vi "RS232_Write-Read String.vi"(4 "Flow Control":u16(ring) items=["None"=0, "RTS-CTS"=256, "DTR-DSR"=512, "XOn-XOff"=1024], 5 "Stop Bits":u8(ring) items=["FT_STOP_BITS_1"=0, "FT_STOP_BITS_2"=2], 6 "Parity":u8(ring) items=["FT_PARITY_NONE", "FT_PARITY_ODD", "FT_PARITY_EVEN", "FT_PARITY_MARK", "FT_PARITY_SPACE"], 7 "Word Length":u8(ring)=8 items=["FT_BITS_7"=7, "FT_BITS_8"=8], 8 "Read Delay (ms)":u32=100, 9 "Write Buffer":string, 10 "Baud Rate":u32=115200, 11 "Device Description":string="TTL232RG-3V3_Application") -> (0 "Bytes Written":u32, 2 "Bytes Read":u32, 3 "Read Buffer Out":string)   [LabVIEW 2018]
panel:
  out "Ok?":bool
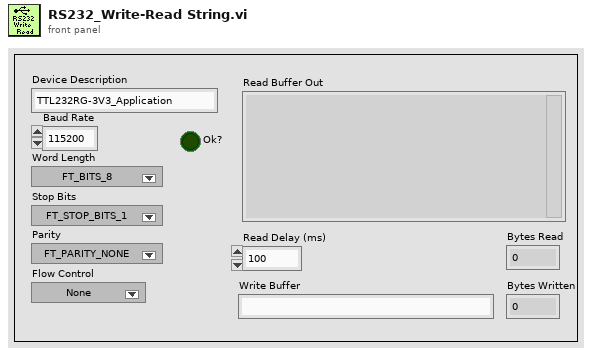
[diagram p1: front panel]
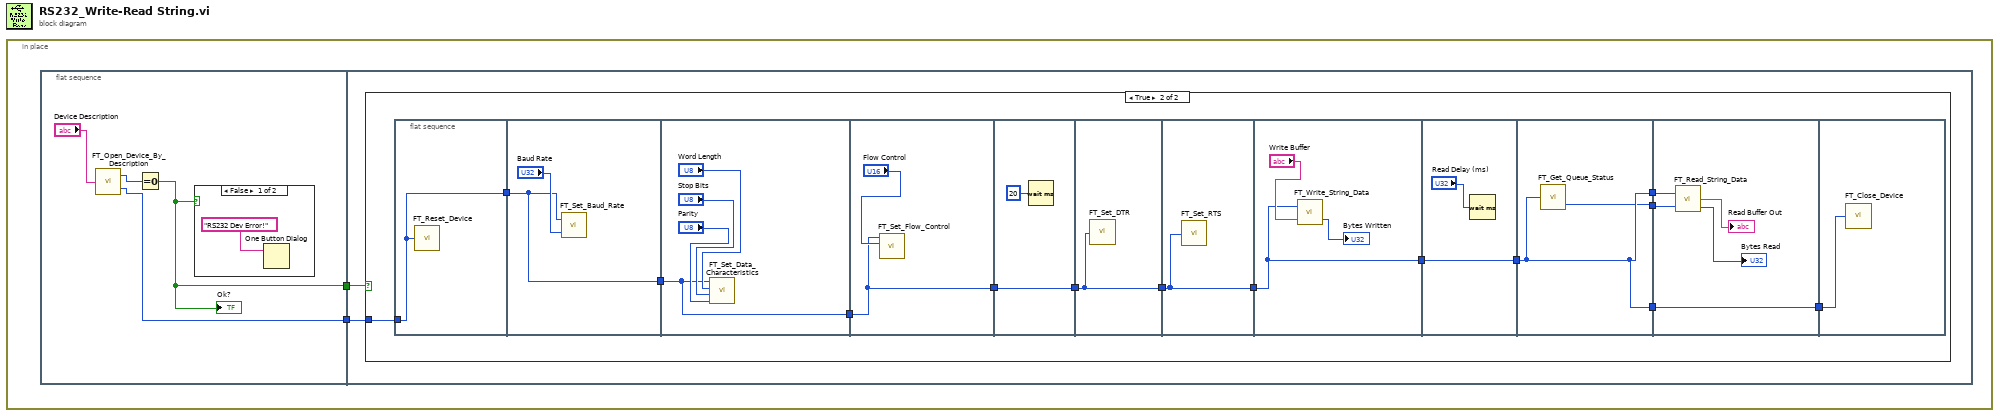
[diagram p0: block diagram]
diagram:
  n1 = in-place {
    n2 = flat-sequence {
      tunnel: [w5] -> w2
      tunnel: [w3] -> w1
      tunnel: w2 -> [w9]
      tunnel: w1 -> [w8]
      frame #0 {
        n3 = call "FT_Open_Device_By_Description.vi"("Device Description"="Device Description") -> ("FT_Status"=w4:u32, "Handle"=w3:u32)
        n4 = Equal To 0?(x=w4) -> (x = 0?=w5:bool)
        "Ok?" <- w5
        n5 = case shown="False" w5 {
          frame False {
            n6 = One Button Dialog(message="RS232 Dev Error!") -> ()  [unwired: 1 in, 1 out]
          }
          frame True {
          }
        }
      }
      frame #1 {
        n7 = case shown="True" w9 {
          tunnel: w8 -> [_ w14]
          frame False {
          }
          frame True {
            n8 = flat-sequence {
              tunnel: [w24] -> w23
              tunnel: w14 -> [w24]
              tunnel: w23 -> [w25]
              tunnel: [w25] -> w22
              tunnel: w22 -> [w27]
              tunnel: [w27] -> w21
              tunnel: w21 -> [w31]
              tunnel: [w31] -> w13
              tunnel: w13 -> [w34]
              tunnel: [w34] -> w12
              tunnel: w12 -> [w35]
              tunnel: [w35] -> w20
              tunnel: w20 -> [w36]
              tunnel: [w36] -> w19
              tunnel: w19 -> [w37]
              tunnel: [w37] -> w11
              tunnel: w11 -> [w41]
              tunnel: [w41] -> w10
              tunnel: w10 -> [w43]
              tunnel: [w42] -> w18
              tunnel: [w43] -> w17
              tunnel: [w43] -> w16
              tunnel: w18 -> [w48]
              tunnel: w17 -> [w47]
              tunnel: w16 -> [w44]
              tunnel: [w44] -> w15
              tunnel: w15 -> [w49]
              frame #0 {
                n9 = call "FT_Reset_Device.vi"("Handle"=w24) -> ()  [unwired: 1 out]
              }
              frame #1 {
                n10 = call "FT_Set_Baud_Rate.vi"("Baud Rate"="Baud Rate", "Handle"=w25) -> ()  [unwired: 1 out]
              }
              frame #2 {
                n11 = call "FT_Set_Data_Characteristics.vi"("Parity"="Parity", "Stop Bits"="Stop Bits", "Word Length"="Word Length", "Handle"=w27) -> ()  [unwired: 1 out]
              }
              frame #3 {
                n12 = call "FT_Set_Flow_Control.vi"("Flow Control"="Flow Control", "Handle"=w31) -> ()  [unwired: 2 in, 1 out]
              }
              frame #4 {
                n13 = Wait (ms)(milliseconds to wait=u32 20) -> ()  [unwired: 1 out]
              }
              frame #5 {
                n14 = call "FT_Set_DTR.vi"("Handle"=w35) -> ()  [unwired: 1 out]
              }
              frame #6 {
                n15 = call "FT_Set_RTS.vi"("Handle"=w36) -> ()  [unwired: 1 out]
              }
              frame #7 {
                n16 = call "FT_Write_String_Data.vi"("Buffer"="Write Buffer", "Handle"=w37) -> ("Bytes Written"=→"Bytes Written":u32)  [unwired: 1 out]
              }
              frame #8 {
                n17 = Wait (ms)(milliseconds to wait="Read Delay (ms)") -> ()  [unwired: 1 out]
              }
              frame #9 {
                n18 = call "FT_Get_Queue_Status.vi"("Handle"=w43) -> ("Bytes Waiting"=w42:u32)  [unwired: 1 out]
              }
              frame #10 {
                n19 = call "FT_Read_String_Data.vi"("Handle"=w47, "Bytes To Read"=w48) -> ("Read Data"=→"Read Buffer Out":string, "Bytes Read"=→"Bytes Read":u32)  [unwired: 1 out]
              }
              frame #11 {
                n20 = call "FT_Close_Device.vi"("Handle"=w49) -> ()  [unwired: 1 out]
              }
            }
          }
        }
      }
    }
  }
